vi "keycommand.vi"(0 "HGF_GPG in":refnum<class "HGF_GPG.lvclass">, 1 "options file":path, 3 "keyringfile":path, 4 "Sec keyringfile":path, 5 "targetfile":path, 7 "error in (no error)":errorcluster, 8 "key-id":string, 9 "SecKey (f)":bool, 10 "Trust DB":path, 12 "Enum":T1(ring), 14 "overwrite? (t)":bool=TRUE) -> (13 "return code":i32, 15 "standard error":string, 16 "data error?":bool, 17 "standard output":string, 18 "dup Trust DB":path, 20 "HGF_GPG out":refnum<class "HGF_GPG.lvclass">, 21 "dup options file":path, 23 "dup keyringfile":path, 24 "dup Sec keyringfile":path, 25 "dup targetfile":path, 27 "error out":errorcluster)   [LabVIEW 2012, in "HGF_GPG.lvlib" / "HGF_GPG.lvclass"]
doc: "Executes following commandline tools of the GnuPG:\ndelete key\nexport key\nimport key"
uses:
  HGF_GPG.lvclass
  HGF_GPG.lvclass/HGF_GPG.ctl
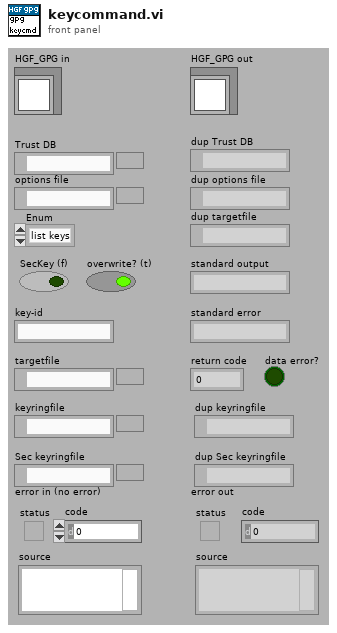
[diagram p1: front panel]
types:
  T1 = enum16{"list keys", "export", "import", "delete"}
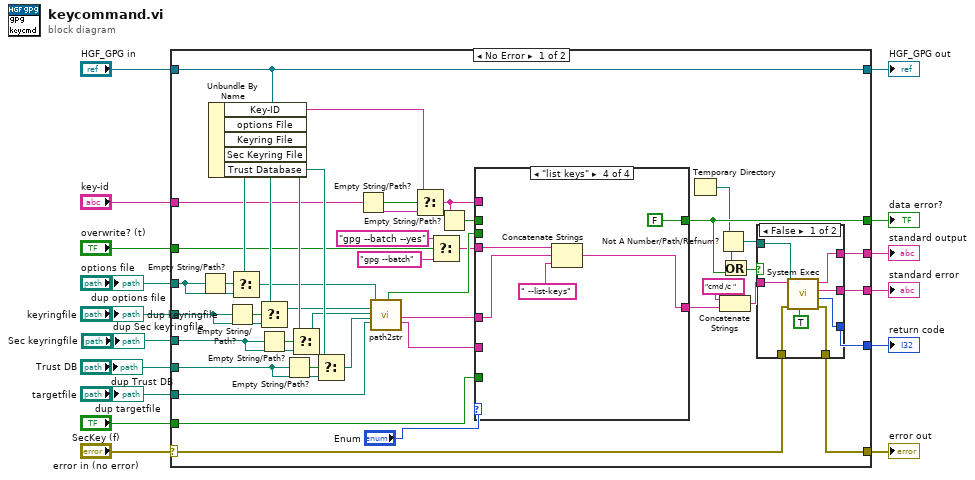
[diagram p0: block diagram]
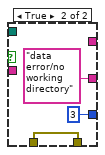
[diagram p2: hidden frame]
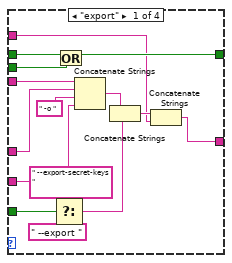
[diagram p3: hidden frame]
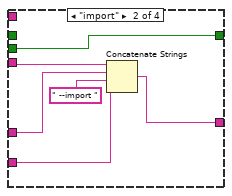
[diagram p4: hidden frame]
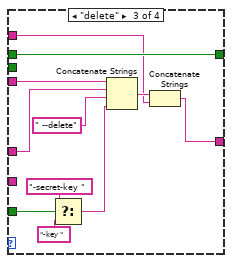
[diagram p5: hidden frame]
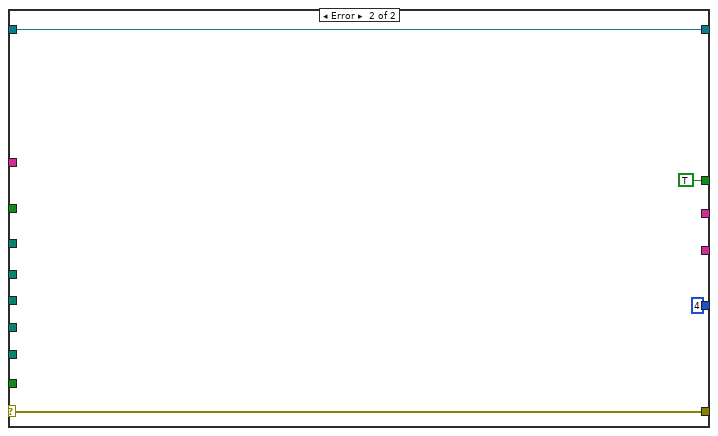
[diagram p6: hidden frame]
diagram:
  n1 = case shown="No Error" "error in (no error)" {
    selector: "error in (no error)" -> [w41 w112]
    tunnel: [w40 w112] -> w15
    tunnel: [w53 w111] -> w13
    tunnel: "HGF_GPG in" -> [w53 w111]
    tunnel: "overwrite? (t)" -> [w54 _]
    tunnel: "key-id" -> [w52 _]
    tunnel: "SecKey (f)" -> [w47 _]
    tunnel: [w42 TRUE] -> w9
    tunnel: [w39 4 ("return code")] -> w6
    tunnel: [w38 _] -> w7
    tunnel: [w37 _] -> w8
    tunnel: "options file" -> [w31 _]
    tunnel: "keyringfile" -> [w28 _]
    tunnel: "targetfile" -> [w24 _]
    tunnel: "Sec keyringfile" -> [w26 _]
    tunnel: "Trust DB" -> [w20 _]
    frame No Error {
      n2 = Empty String/Path?(string/path=w31) -> (empty?=w32:bool)
      n3 = Unbundle By Name(w53) -> ("Key-ID"=w51:string, "options File"=w56:path, "Keyring File"=w57:path, "Sec Keyring File"=w59:path, "Trust Database"=w60:path)
      n4 = Empty String/Path?(string/path=w28) -> (empty?=w29:bool)
      n5 = Select(t=w56, s=w32, f=w31) -> (s? t:f=w30:path)
      n6 = Select(t=w57, s=w29, f=w28) -> (s? t:f=w23:path)
      n7 = Empty String/Path?(string/path=w26) -> (empty?=w27:bool)
      n8 = Empty String/Path?(string/path=w20) -> (empty?=w21:bool)
      n9 = Select(t=w59, s=w27, f=w26) -> (s? t:f=w22:path)
      n10 = Select(t=w60, s=w21, f=w20) -> (s? t:f=w19:path)
      n11 = Empty String/Path?(string/path=w52) -> (empty?=w50:bool)
      n12 = call "path2str.vi"("options file"=w30, "keyringfile"=w23, "Sec keyringfile"=w22, "Trust DB"=w19, "targetfile"=w24) -> ("tf NaPath"=w58:bool, "opt/keyr/seckeyr/trusdb"=w18:string, "targetfile path"=w25:string)  [unwired: 1 in, 11 out]
      n13 = Select(t=w51, s=w50, f=w52) -> (s? t:f=w46:string)
      n14 = Select(t="gpg --batch --yes", s=w54, f="gpg --batch") -> (s? t:f=w48:string)
      n15 = Empty String/Path?(string/path=w46) -> (empty?=w45:bool)
      n16 = case shown="\"list keys\"" "Enum" {
        tunnel: w46 -> [w75 _ w95 _]
        tunnel: w48 -> [w86 w92 w102 w108]
        tunnel: w47 -> [w83 _ w97 _]
        tunnel: w58 -> [w81 w91 _ _]
        tunnel: w45 -> [w82 _ w103 _]
        tunnel: [w80 w91 w103 FALSE ("tf NaPath")] -> w42
        tunnel: [w76 w90 w96 w104] -> w35
        tunnel: w25 -> [w73 w88 _ _]
        tunnel: w18 -> [w72 w87 w93 w107]
        frame "export" {
          n17 = Select(t=" --export-secret-keys ", s=w83, f=" --export ") -> (s? t:f=w79:string)
          n18 = Or(x=w82, y=w81) -> (x .or. y?=w80:bool)
          n19 = Concatenate Strings(w86, w72, " -o ", w73) -> (w78:string)
          n20 = Concatenate Strings(w78, w79) -> (w77:string)
          n21 = Concatenate Strings(w77, w75) -> (w76:string)
        }
        frame "import" {
          n22 = Concatenate Strings(w92, w87, " --import ", w88) -> (w90:string)
        }
        frame "delete" {
          n23 = Select(t="-secret-key ", s=w97, f="-key ") -> (s? t:f=w99:string)
          n24 = Concatenate Strings(w102, w93, " --delete", w99) -> (w98:string)
          n25 = Concatenate Strings(w98, w95) -> (w96:string)
        }
        frame "list keys" {
          n26 = Concatenate Strings(w108, w107, " --list-keys" ("string")) -> (w104:string)
        }
      }
      n27 = Temporary Directory() -> (w17:path)
      n28 = Not A Number/Path/Refnum?(number/path/refnum=w17) -> (NaN/Path/Refnum?=w44:bool)
      n29 = Concatenate Strings("cmd /c " ("string"), w35) -> (w36:string)
      n30 = Or(x=w44, y=w42) -> (x .or. y?=w43:bool)
      n31 = case shown="False" w43 {
        tunnel: w41 -> [w67 w71]
        tunnel: [w66 w71] -> w40
        tunnel: w17 -> [w65 _]
        tunnel: w36 -> [w64 _]
        tunnel: [w63 _] -> w37
        tunnel: [w62 "data error/no working directory" ("standard error")] -> w38
        tunnel: [w61 3 ("return code")] -> w39
        frame False {
          n32 = call <vilib>:"System Exec.vi"("run minimized? (F)"=TRUE, "error in (no error)"=w67, "working directory"=w65, "command line"=w64) -> ("error out"=w66:errorcluster, "return code"=w61:i32, "standard error"=w62:string, "standard output"=w63:string)  [unwired: 2 in, 2 out]
        }
        frame True {
        }
      }
    }
    frame Error {
    }
  }
  "error out" <- w15
  "HGF_GPG out" <- w13
  "data error?" <- w9
  "standard output" <- w8
  "standard error" <- w7
  "return code" <- w6
  "dup targetfile" <- "targetfile"
  "dup keyringfile" <- "keyringfile"
  "dup options file" <- "options file"
  "dup Sec keyringfile" <- "Sec keyringfile"
  "dup Trust DB" <- "Trust DB"
